vi "TakeGraphsScreenshot.vi"(6 "DefaultFolderName(Data)":string="Data", 7 "Prompt":string, 8 "ErrorIn":errorcluster, 10 "DefaultName":string, 11 "GraphsTabReference":refnum<vi>) -> (0 "ErrorOut":errorcluster)   [LabVIEW 2016]
doc: "Save graphs screenshot to an image files."
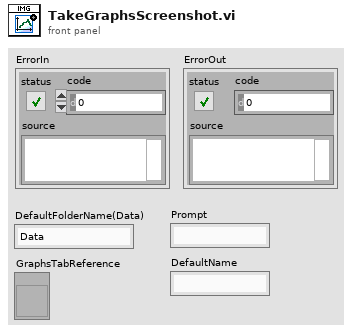
[diagram p1: front panel]
types:
  T1 = typedef "imagedata.ctl" = cluster{"image type":i32, "image depth":i32, "image":u8[], "mask":u8[], "colors":u32[], "Rectangle":cluster{"left":i16, "top":i16, "right":i16, "bottom":i16}}
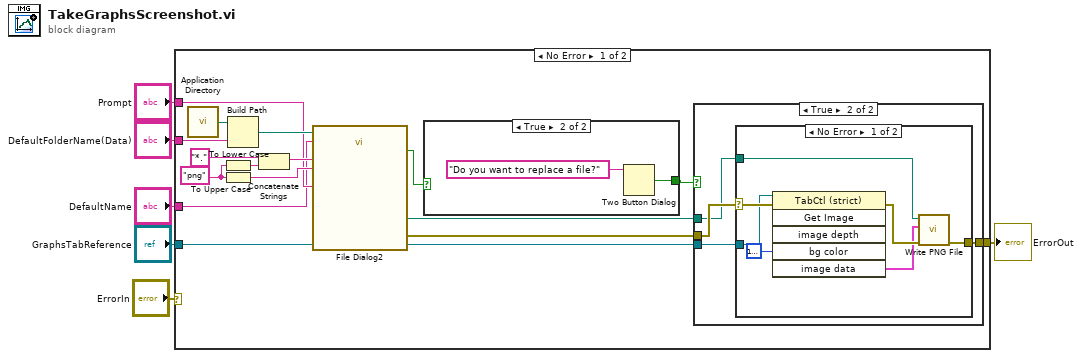
[diagram p0: block diagram]
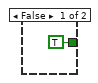
[diagram p4: hidden frame]
diagram:
  n1 = case shown="No Error" "ErrorIn" {
    selector: "ErrorIn" -> [_ w39]
    tunnel: [w22 w39] -> w6
    tunnel: "GraphsTabReference" -> [w21 _]
    tunnel: "DefaultFolderName(Data)" -> [w12 _]
    tunnel: "Prompt" -> [w8 _]
    tunnel: "DefaultName" -> [w7 _]
    frame No Error {
      w14 = "png" ("string")
      n2 = call <vilib>:"Application Directory.vi"() -> ("Application Directory"=w20:path)
      n3 = To Lower Case(string=w14) -> (all lower case string=w17:string)
      n4 = To Upper Case(1:w14) -> (0:w18:string)
      n5 = Build Path(base path=w20, name or relative path=w12) -> (appended path=w19:path)
      n6 = Concatenate Strings("*." ("string"), w17) -> (w15:string)
      n7 = call "File Dialog2"("start path"=w19, "prompt"=w8, "default name"=w7, "pattern (all files)"=w15, "pattern label"=w18) -> ("selected path"=w9:path, "exists"=w13:bool, "error out"=w10:errorcluster)  [unwired: 7 in, 1 out]
      n8 = case shown="True" w13 {
        tunnel: [TRUE ("T button?") w38] -> w11
        frame False {
        }
        frame True {
          n9 = Two Button Dialog(message="Do you want to replace a file?") -> (T button?=w38:bool)  [unwired: 2 in]
        }
      }
      n10 = case shown="True" w11 {
        tunnel: [w23 w27] -> w22
        tunnel: w21 -> [_ w26]
        tunnel: w10 -> [w23 w25]
        tunnel: w9 -> [_ w24]
        frame False {
        }
        frame True {
          n11 = case shown="No Error" w25 {
            selector: w25 -> [w33 w35]
            tunnel: [w34 w35] -> w27
            tunnel: w24 -> [w28 _]
            tunnel: w26 -> [w32 _]
            frame No Error {
              n12 = invoke on="Invoke Node" class="TabCtl (strict)" method="Get Image"(reference=w32, error in=w33, "bg color"=u32 16777226) -> (error out=w31:errorcluster, "image data"=w30:T1)  [unwired: 3 in, 4 out]
              n13 = call <vilib>:"Write PNG File.vi"("error in (no error)"=w31, "image data"=w30, "path to PNG file"=w28) -> ("error out"=w34:errorcluster)  [unwired: 7 in, 1 out]
            }
            frame Error {
            }
          }
        }
      }
    }
    frame Error {
    }
  }
  "ErrorOut" <- w6
